vi "Initialize Attributes.vi"(8 "error in (no error)":errorcluster, 10 "Attribute Data":variant, 11 "CS++DCPwr in":refnum<class "CS++DCPwr.lvclass">) -> (0 "error out":errorcluster, 2 "Found?":bool, 3 "CS++DCPwr out":refnum<class "CS++DCPwr.lvclass">)   [LabVIEW 2014, in "CS++DCPwr.lvlib" / "CS++DCPwr.lvclass"]
doc: "Initialize object attribute.\n\nUnique resources should be allocated elsewhere!"
uses:
  CS++DCPwr.lvclass
  CSPP_Core/Classes/CS++BaseClasses/Factory/CS++Factory.lvclass
  CSPP_Core/Actors/CS++BaseActor/CS++BaseActor.lvclass
  CSPP_Core/Libraries/Utilities/CS++Utilities.lvlib
  CSPP_Core/Actors/CS++DeviceActor/CS++DeviceActor.lvclass
  CSPP_Core/Classes/CS++ProcessVariables/ProcessVariable/PV.lvclass
  CSPP_Core/Classes/CS++ProcessVariables/CS++ProcessVariables.lvlib
  PV-Enum.ctl
panel:
  in  "PV-Enum":T1
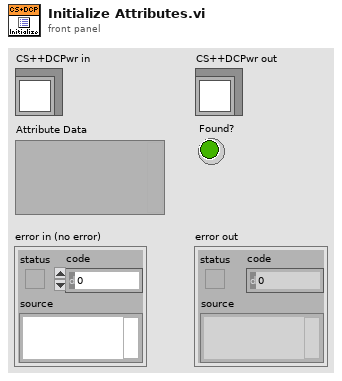
[diagram p1: front panel]
types:
  T1 = typedef "CS++DCPwr.lvlib/CS++DCPwr.lvclass/PV-Enum.ctl" = enum16{"CurrentLimit", "MaxCurrentLimit", "MaxVoltageLevel", "Measure-A", "Measure-V", "OVPLimit", "Range", "TriggerCurrentLimit", "TriggerVoltageLevel", "VoltageLevel", "Behavior", "DesiredOutputState", "RangeType", "TriggerSource", "InState", "OutputEnable", "OVPEnabled"}
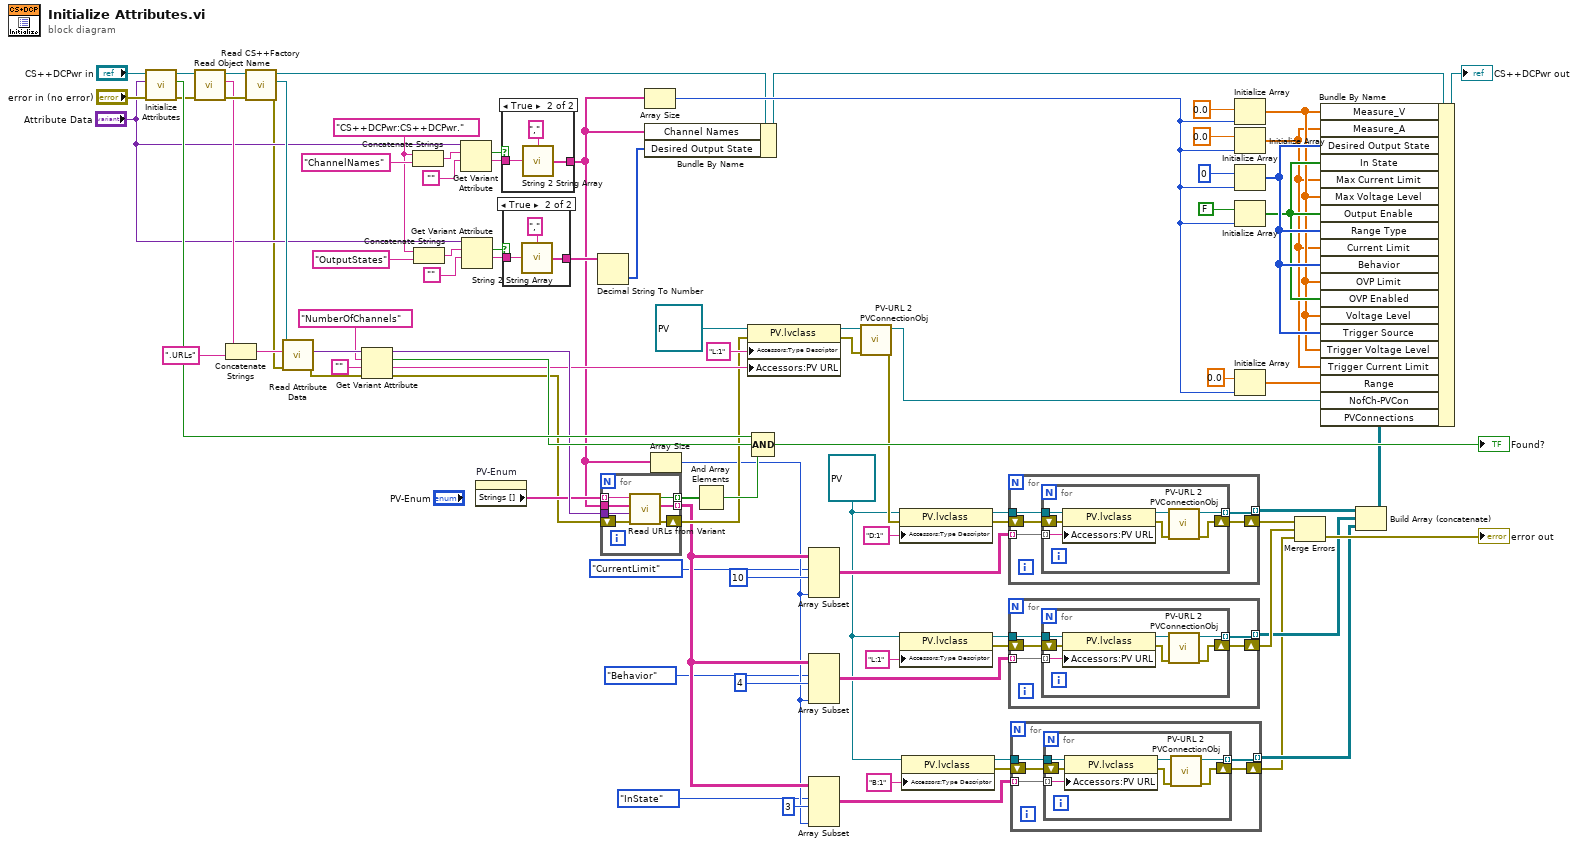
[diagram p0: block diagram]
diagram:
  w11 = refnum<class "PV.lvclass"> refnum ("CS++ProcessVariables.lvlib:PV.lvclass")
  w68 = "CS++DCPwr:CS++DCPwr."
  n1 = call-parent "Initialize Attributes.vi"("error in (no error)"="error in (no error)", "Attribute Data"="Attribute Data", "CS++DeviceActor in"="CS++DCPwr in") -> ("error out"=w81:errorcluster, "Found?"=w83:bool, "CS++DeviceActor out"=w82:refnum<class "CS++DCPwr.lvclass">)  [unwired: 6 in]
  n2 = call "Read Object Name.vi"("error in (no error)"=w81, "CS++BaseActor in"=w82) -> ("error out"=w84:errorcluster, "Object Name"=w80:string, "CS++BaseActor out"=w85:refnum<class "CS++DCPwr.lvclass">)  [unwired: 7 in]
  n3 = Concatenate Strings(w80, ".URLs" ("string")) -> (w86:string)
  n4 = call "Read CS++Factory.vi"("error in (no error)"=w84, "CS++BaseActor in"=w85) -> ("error out"=w62:errorcluster, "CS++Factory"=w79:refnum<class "CS++Factory.lvclass">, "CS++BaseActor out"=w44:refnum<class "CS++DCPwr.lvclass">)  [unwired: 7 in]
  n5 = call-dynamic "Read Attribute Data.vi"("error in (no error)"=w62, "Object Name"=w86, "CS++Factory in"=w79) -> ("error out"=w63:errorcluster, "Attribute Data"=w61:variant)  [unwired: 6 in, 1 out]
  n6 = Get Variant Attribute(Variant=w61, name="NumberOfChannels" ("string"), default value (empty Variant)="", error in=w63) -> (duplicate Variant=w57:variant, found=w58:bool, value=w33:string, error out=w41:errorcluster)
  n7 = Concatenate Strings(w68, "ChannelNames" ("string")) -> (w77:string)
  n8 = Concatenate Strings(w68, "OutputStates" ("string")) -> (w70:string)
  n9 = Get Variant Attribute(Variant="Attribute Data", name=w77, default value (empty Variant)="") -> (found=w74:bool, value=w75:string)  [unwired: 1 in, 2 out]
  n10 = Get Variant Attribute(Variant="Attribute Data", name=w70, default value (empty Variant)="") -> (found=w73:bool, value=w72:string)  [unwired: 1 in, 2 out]
  n11 = property on="PV-Enum" class="Enum (strict)"() -> ("Strings []"=w43:string[])  [unwired: 2 in, 2 out]
  n12 = case shown="True" w74 {
    tunnel: w75 -> [_ w91]
    tunnel: [_ w90] -> w8
    frame False {
    }
    frame True {
      n13 = call "String 2 String Array.vi"("String"=w91, "Delimiter (\",\")"="," ("Delimiter (\",\")")) -> ("Substrings"=w90:string[])
    }
  }
  n14 = case shown="True" w73 {
    tunnel: w72 -> [_ w94]
    tunnel: [_ w93] -> w67
    frame False {
    }
    frame True {
      n15 = call "String 2 String Array.vi"("String"=w94, "Delimiter (\",\")"="," ("Delimiter (\",\")")) -> ("Substrings"=w93:string[])
    }
  }
  n16 = Decimal String To Number(string=w67) -> (number=w64:i32[])  [unwired: 2 in, 1 out]
  n17 = for {
    tunnel: w43 -> [w102] mode=indexing
    tunnel: [w101] -> w65 mode=indexing
    tunnel: w57 -> [w99]
    tunnel: w8 -> [w98]
    tunnel: [w97] -> w12 mode=indexing
    shift-right: [w100] -> w30
    shift-left: w41 -> [w96]
    n18 = call "Read URLs from Variant.vi"("Error In"=w96, "URL Section Data"=w99, "Channel Names"=w98, "URL Prefix"=w102) -> ("Error Out"=w100:errorcluster, "URLs"=w97:string[], "Found?"=w101:bool)  [unwired: 5 in]
  }
  n19 = Array Size(array=w8) -> (size(s)=w53:i32)
  n20 = Bundle By Name(cluster=w44, "Channel Names"=w8, "Desired Output State"=w64) -> (w26:refnum<class "CS++DCPwr.lvclass">)
  n21 = Array Size(array=w8) -> (size(s)=w4:i32)
  n22 = And Array Elements(Boolean array=w65) -> (logical AND=w42:bool)
  n23 = property class="PV.lvclass"(reference=refnum<class "PV.lvclass"> refnum ("CS++ProcessVariables.lvlib:PV.lvclass"), error in=w30, "Accessors:Type Descriptor"="L:1" ("Type Descriptor"), "Accessors:PV URL"=w33) -> (reference out=w31:refnum<class "PV.lvclass">, error out=w32:errorcluster)
  n24 = Compound Arithmetic op=AND(w83, w58, w42) -> (→"Found?":bool)
  n25 = Array Subset(array=w12, index (row)=PV-Enum."CurrentLimit" ("PV-Enum"), length (row)=10 ("length"), length (col)=w4) -> (w37:string[][])  [unwired: 1 in]
  n26 = Array Subset(array=w12, index (row)=PV-Enum."Behavior" ("PV-Enum"), length (row)=4 ("length"), length (col)=w4) -> (w17:string[][])  [unwired: 1 in]
  n27 = Array Subset(array=w12, index (row)=PV-Enum."InState" ("PV-Enum"), length (row)=3 ("length"), length (col)=w4) -> (w16:string[][])  [unwired: 1 in]
  n28 = call "PV-URL 2 PVConnectionObj.vi"("Error In"=w32, "PV"=w31) -> ("Error Out"=w29:errorcluster, "PVConnection"=w27:refnum<class "PVConnection.lvclass">)  [unwired: 7 in, 1 out]
  n29 = property class="PV.lvclass"(reference=w11, error in=w29, "Accessors:Type Descriptor"="D:1" ("Type Descriptor")) -> (reference out=w35:refnum<class "PV.lvclass">, error out=w34:errorcluster)
  n30 = property class="PV.lvclass"(reference=w11, "Accessors:Type Descriptor"="L:1" ("Type Descriptor")) -> (reference out=w22:refnum<class "PV.lvclass">, error out=w23:errorcluster)  [unwired: 1 in]
  n31 = property class="PV.lvclass"(reference=w11, "Accessors:Type Descriptor"="B:1" ("Type Descriptor")) -> (reference out=w14:refnum<class "PV.lvclass">, error out=w13:errorcluster)  [unwired: 1 in]
  n32 = for {
    tunnel: w35 -> [w107]
    tunnel: w37 -> [w106] mode=indexing
    tunnel: [w105] -> w25 mode=indexing
    shift-right: [w104] -> w28
    shift-left: w34 -> [w103]
    n33 = for {
      tunnel: w107 -> [w113]
      tunnel: w106 -> [w112] mode=indexing
      tunnel: [w111] -> w105 mode=indexing
      shift-right: [w110] -> w104
      shift-left: w103 -> [w108]
      n34 = property class="PV.lvclass"(reference=w113, error in=w108, "Accessors:PV URL"=w112) -> (reference out=w114:refnum<class "PV.lvclass">, error out=w109:errorcluster)
      n35 = call "PV-URL 2 PVConnectionObj.vi"("Error In"=w109, "PV"=w114) -> ("Error Out"=w110:errorcluster, "PVConnection"=w111:refnum<class "PVConnection.lvclass">)  [unwired: 7 in, 1 out]
    }
  }
  n36 = for {
    tunnel: w22 -> [w119]
    tunnel: w17 -> [w118] mode=indexing
    tunnel: [w117] -> w18 mode=indexing
    shift-right: [w116] -> w19
    shift-left: w23 -> [w115]
    n37 = for {
      tunnel: w119 -> [w125]
      tunnel: w118 -> [w124] mode=indexing
      tunnel: [w123] -> w117 mode=indexing
      shift-right: [w122] -> w116
      shift-left: w115 -> [w120]
      n38 = property class="PV.lvclass"(reference=w125, error in=w120, "Accessors:PV URL"=w124) -> (reference out=w126:refnum<class "PV.lvclass">, error out=w121:errorcluster)
      n39 = call "PV-URL 2 PVConnectionObj.vi"("Error In"=w121, "PV"=w126) -> ("Error Out"=w122:errorcluster, "PVConnection"=w123:refnum<class "PVConnection.lvclass">)  [unwired: 7 in, 1 out]
    }
  }
  n40 = for {
    tunnel: w14 -> [w131]
    tunnel: w16 -> [w130] mode=indexing
    tunnel: [w129] -> w10 mode=indexing
    shift-right: [w128] -> w9
    shift-left: w13 -> [w127]
    n41 = for {
      tunnel: w131 -> [w137]
      tunnel: w130 -> [w136] mode=indexing
      tunnel: [w135] -> w129 mode=indexing
      shift-right: [w134] -> w128
      shift-left: w127 -> [w132]
      n42 = property class="PV.lvclass"(reference=w137, error in=w132, "Accessors:PV URL"=w136) -> (reference out=w138:refnum<class "PV.lvclass">, error out=w133:errorcluster)
      n43 = call "PV-URL 2 PVConnectionObj.vi"("Error In"=w133, "PV"=w138) -> ("Error Out"=w134:errorcluster, "PVConnection"=w135:refnum<class "PVConnection.lvclass">)  [unwired: 7 in, 1 out]
    }
  }
  n44 = Initialize Array(dbl[unit] 0.0 ("measurement"), w53) -> (w48:dbl[unit][])
  n45 = Initialize Array(dbl[unit] 0.0 ("measurement"), w53) -> (w47:dbl[unit][])
  n46 = Initialize Array(0 ("output state (Constant Voltage)"), w53) -> (w50:i32[])
  n47 = Initialize Array(FALSE ("in state"), w53) -> (w49:bool[])
  n48 = Initialize Array(0.0 ("range (0.0)"), w53) -> (w45:dbl[])
  n49 = Merge Errors(w28, w19, w9) -> (→"error out":errorcluster)
  n50 = Build Array (concatenate)(w25, w18, w10) -> (w24:refnum<class "PVConnection.lvclass">[][])
  n51 = Bundle By Name(cluster=w26, "Measure_V"=w48, "Measure_A"=w47, "Desired Output State"=w50, "In State"=w49, "Max Current Limit"=w47, "Max Voltage Level"=w48, "Output Enable"=w49, "Range Type"=w50, "Current Limit"=w47, "Behavior"=w50, "OVP Limit"=w48, "OVP Enabled"=w49, "Voltage Level"=w48, "Trigger Source"=w50, "Trigger Voltage Level"=w48, "Trigger Current Limit"=w47, "Range"=w45, "NofCh-PVCon"=w27, "PVConnections"=w24) -> (→"CS++DCPwr out":refnum<class "CS++DCPwr.lvclass">)
